vi "S2C_FORNAX_Proc_CreateAlarmQ.vi"(8 "Error In":errorcluster) -> (0 "Error Out":errorcluster)   [LabVIEW 2015]
doc: "Reads the data contained within the Fornax Commands file and loads the data into the Fornax global variables."
uses:
  S2C_FORNAX_Proc_Globals.vi
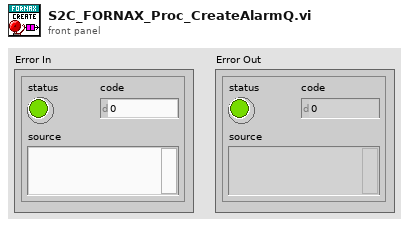
[diagram p1: front panel]
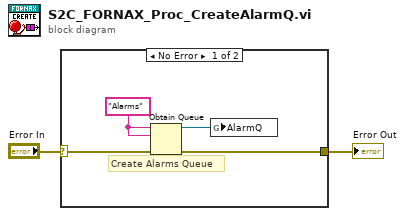
[diagram p0: block diagram]
diagram:
  n1 = case shown="No Error" "Error In" {
    selector: "Error In" -> [w4 w7]
    tunnel: [w3 w7] -> w1
    frame No Error {
      w6 = "Alarms"
      # "Create Alarms Queue"
      n2 = Obtain Queue(name (unnamed)=w6, element data type=w6, error in (no error)=w4) -> (queue out=w5:refnum<queue>, error out=w3:errorcluster)  [unwired: 2 in, 1 out]
      n3 = global write "S2C_FORNAX_Proc_Globals.vi" "AlarmQ"(w5) -> ()
    }
    frame Error {
    }
  }
  "Error Out" <- w1
